vi "Set Bitrate Adapting.vi"(8 "error in":errorcluster, 10 "Enable":bool, 11 "TPCANHandle in":T2=81 items=["PCAN_NONEBUS"=0, "PCAN_USBBUS1"=81, "PCAN_USBBUS2"=82, "PCAN_USBBUS3"=83, "PCAN_USBBUS4"=84, "PCAN_USBBUS5"=85, "PCAN_USBBUS6"=86, "PCAN_USBBUS7"=87, "PCAN_USBBUS8"=88, "PCAN_USBBUS9"=1289, "PCAN_USBBUS10"=1290, "PCAN_USBBUS11"=1291, "PCAN_USBBUS12"=1292, "PCAN_USBBUS13"=1293, "PCAN_USBBUS14"=1294, "PCAN_USBBUS15"=1295, "PCAN_USBBUS16"=1296]) -> (0 "error out":errorcluster, 3 "TPCANHandle out":T2=81 items=["PCAN_NONEBUS"=0, "PCAN_USBBUS1"=81, "PCAN_USBBUS2"=82, "PCAN_USBBUS3"=83, "PCAN_USBBUS4"=84, "PCAN_USBBUS5"=85, "PCAN_USBBUS6"=86, "PCAN_USBBUS7"=87, "PCAN_USBBUS8"=88, "PCAN_USBBUS9"=1289, "PCAN_USBBUS10"=1290, "PCAN_USBBUS11"=1291, "PCAN_USBBUS12"=1292, "PCAN_USBBUS13"=1293, "PCAN_USBBUS14"=1294, "PCAN_USBBUS15"=1295, "PCAN_USBBUS16"=1296], 5 "TPCANStatus":T1 items=["PCAN_ERROR_OK"=0, "PCAN_ERROR_XMTFULL"=1, "PCAN_ERROR_OVERRUN"=2, "PCAN_ERROR_BUSLIGHT"=4, "PCAN_ERROR_BUSHEAVY"=8, "PCAN_ERROR_BUSPASSIVE"=262144, "PCAN_ERROR_BUSOFF"=16, "PCAN_ERROR_QRCVEMPTY"=32, "PCAN_ERROR_QOVERRUN"=64, "PCAN_ERROR_QXMTFULL"=128, "PCAN_ERROR_REGTEST"=256, "PCAN_ERROR_NODRIVER"=512, "PCAN_ERROR_HWINUSE"=1024, "PCAN_ERROR_NETINUSE"=2048, "PCAN_ERROR_ILLHW"=5120, "PCAN_ERROR_ILLNET"=6144, "PCAN_ERROR_ILLCLIENT"=7168, "PCAN_ERROR_RESOURCE"=8192, "PCAN_ERROR_ILLPARAMTYPE"=16384, "PCAN_ERROR_ILLPARAMVAL"=32768, "PCAN_ERROR_UNKNOWN"=65536, "PCAN_ERROR_ILLDATA"=131072, "PCAN_ERROR_ILLMODE"=524288, "PCAN_ERROR_CAUTION"=33554432, "PCAN_ERROR_INITIALIZE"=67108864, "PCAN_ERROR_ILLOPERATION"=134217728])   [LabVIEW 2020, in "PCANBasic.lvlib"]
doc: "This parameter allows the user to connect to an active PCAN-Channel when the bit rate used\nis unknown. When this mode is set, PCAN-Basic will try first to use the bit rate given as\nparameter in the initialization process; if the channel has a different bit rate configured, then\nthe new connection will use the configured bit rate and the initialization function will return\na warning value, indicating that the used bit rate differs from the given one.\nThis parameter is a so called “pre-initialized only” parameter, which means that it can be\nonly set before a PCAN-Channel is initialized.\n\nThe default state of the Bitrate-Adapting mode is deactivated (PCAN_PARAMETER_OFF). This\nparameter has effect only at initialize time. It cannot be set after activating a channel. The\nparameter returns to its default value after calling the initialize/InitializeFD function."
uses:
  PCANBasic.lvlib
  TPCANParameter.ctl
  TPCANHandle.ctl
  TPCANStatus.ctl
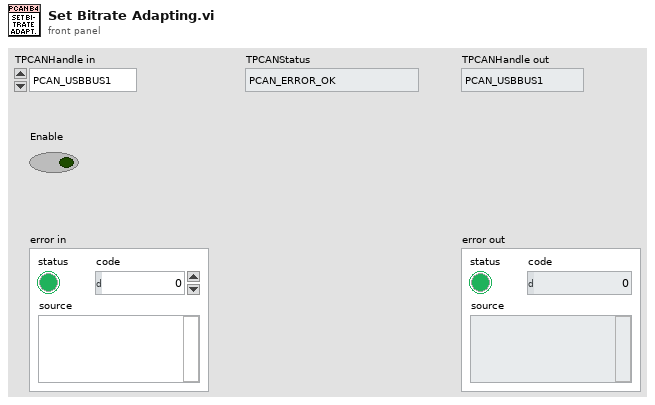
[diagram p1: front panel]
types:
  T1 = typedef "PCANBasic.lvlib/TPCANStatus.ctl" = u32
  T2 = typedef "PCANBasic.lvlib/TPCANHandle.ctl" = u16
  T3 = typedef "PCANBasic.lvlib/TPCANParameter.ctl" = enum8{"Unknown", "PCAN_DEVICE_ID", "PCAN_5VOLTS_POWER", "PCAN_RECEIVE_EVENT", "PCAN_MESSAGE_FILTER", "PCAN_API_VERSION", "PCAN_CHANNEL_VERSION", "PCAN_BUSOFF_AUTORESET", "PCAN_LISTEN_ONLY", "PCAN_LOG_LOCATION", "PCAN_LOG_STATUS", "PCAN_LOG_CONFIGURE", "PCAN_LOG_TEXT", "PCAN_CHANNEL_CONDITION", "PCAN_HARDWARE_NAME", "PCAN_RECEIVE_STATUS", "PCAN_CONTROLLER_NUMBER", "PCAN_TRACE_LOCATION", "PCAN_TRACE_STATUS", "PCAN_TRACE_SIZE", "PCAN_TRACE_CONFIGURE", "PCAN_CHANNEL_IDENTIFYING", "PCAN_CHANNEL_FEATURES", "PCAN_BITRATE_ADAPTING", "PCAN_BITRATE_INFO", "PCAN_BITRATE_INFO_FD", "PCAN_BUSSPEED_NOMINAL", "PCAN_BUSSPEED_DATA", "PCAN_IP_ADDRESS", "PCAN_LAN_SERVICE_STATUS", "PCAN_ALLOW_STATUS_FRAMES", "PCAN_ALLOW_RTR_FRAMES", "PCAN_ALLOW_ERROR_FRAMES", "PCAN_INTERFRAME_DELAY", "PCAN_ACCEPTANCE_FILTER_11BIT", "PCAN_ACCEPTANCE_FILTER_29BIT", "PCAN_IO_DIGITAL_CONFIGURATION", "PCAN_IO_DIGITAL_VALUE", "PCAN_IO_DIGITAL_SET", "PCAN_IO_DIGITAL_CLEAR", "PCAN_IO_ANALOG_VALUE", "PCAN_FIRMWARE_VERSION", "PCAN_ATTACHED_CHANNELS_COUNT", "PCAN_ATTACHED_CHANNELS", "PCAN_ALLOW_ECHO_FRAMES", "PCAN_DEVICE_PART_NUMBER", "PCAN_HARD_RESET_STATUS", "PCAN_LAN_CHANNEL_DIRECTION", "PCAN_DEVICE_GUID"}
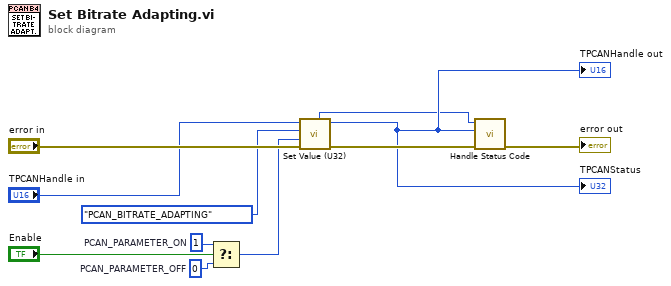
[diagram p0: block diagram]
diagram:
  w8 = u32 0  # PCAN_PARAMETER_OFF
  w9 = u32 1  # PCAN_PARAMETER_ON
  n1 = Select(t=w9, s="Enable", f=w8) -> (s? t:f=w4:u32)
  n2 = call "Set Value (U32).vi"("error in"="error in", "Value"=w4, "TPCANParameter"=TPCANParameter."PCAN_BITRATE_ADAPTING", "TPCANHandle in"="TPCANHandle in") -> ("error out"=w6:errorcluster, "TPCANHandle out"=w2:T2, "TPCANStatus"=w1:u32)  [unwired: 5 in]
  "TPCANHandle out" <- w2
  "TPCANStatus" <- w2
  n3 = call "Handle Status Code.vi"("error in"=w6, "TPCANHandle"=w2, "TPCANStatus"=w1) -> ("error out"=→"error out":errorcluster)  [unwired: 8 in]
